vi "Read Languages.vi"(8 "error in (no error)":errorcluster, 11 "Menu Data in":refnum<class "Menu Data.lvclass">) -> (0 "error out":errorcluster, 2 "Languages":T1[](array[typedef]), 3 "Menu Data out":refnum<class "Menu Data.lvclass">)   [LabVIEW 2013, in "SET Project Data.lvlib" / "Menu Data.lvclass"]
uses:
  Menu Data.lvclass
  Types/ProjFile_Language Entry.ctl
  Menu Data.lvclass/Menu Data.ctl
  Resource Data Class/Resource Data.lvclass/Resource Data.ctl
  Resource Data Class/Resource Data.lvclass
  SET Project Data.lvlib
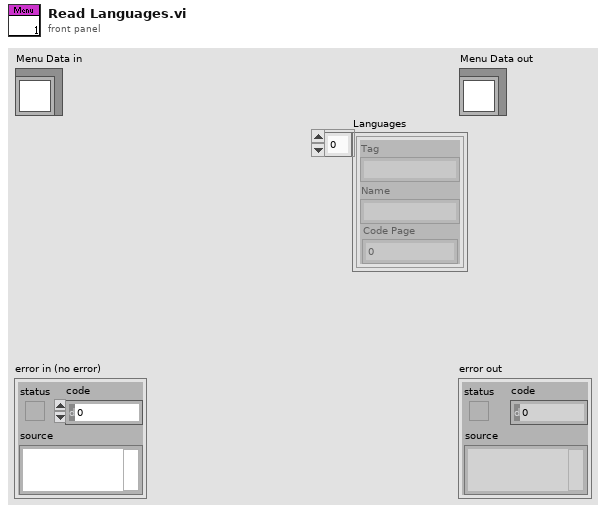
[diagram p1: front panel]
types:
  T1 = typedef "SET Project Data.lvlib/ProjFile_Language Entry.ctl" = cluster{"Tag":string, "Name":string, "Code Page":u16}
  T2 = typedef "SET Project Data.lvlib/ProjFile_Language Data.ctl" = cluster{"Tag":string, "Name":string, "Code Page":u16}
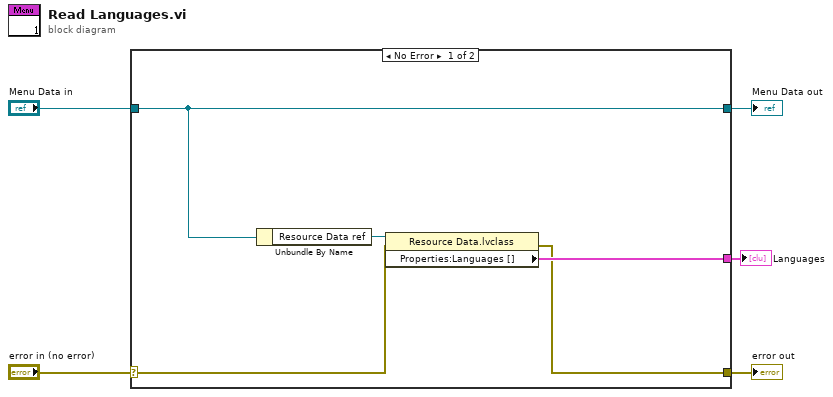
[diagram p0: block diagram]
diagram:
  n1 = case shown="No Error" "error in (no error)" {
    selector: "error in (no error)" -> [w7 w12]
    tunnel: [w6 w12] -> w4
    tunnel: [w10 w11] -> w2
    tunnel: "Menu Data in" -> [w10 w11]
    tunnel: [w8 _] -> w1
    frame No Error {
      n2 = Unbundle By Name(w10) -> ("Resource Data ref"=w9:refnum<data-value>)
      n3 = property class="Resource Data.lvclass"(reference=w9, error in=w7) -> (error out=w6:errorcluster, "Properties:Languages []"=w8:T2[])  [unwired: 1 out]
    }
    frame Error {
    }
  }
  "error out" <- w4
  "Menu Data out" <- w2
  "Languages" <- w1
